vi "Report_Status_Channels.vi"(8 "error in (no error)":errorcluster, 9 "FIFO Indexes":i32[](array[numeric]), 10 "Iteration Duration (us)":u32, 11 "Data (in)":dbl[](array[numeric])) -> (0 "error out":errorcluster, 3 "Data (out)":dbl[](array[numeric]))   [LabVIEW 2019, in "Ballard Arinc-429 Engine.lvlib"]
uses:
  Ballard Arinc-429 Engine.lvlib
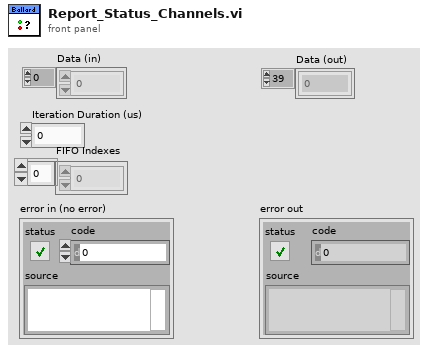
[diagram p1: front panel]
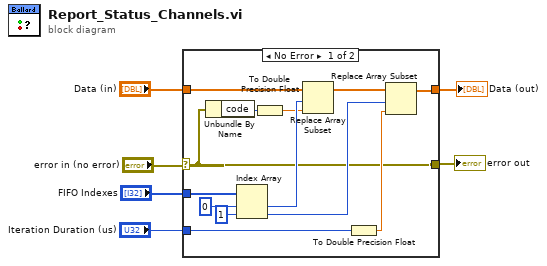
[diagram p0: block diagram]
diagram:
  n1 = case shown="No Error" "error in (no error)" {
    selector: "error in (no error)" -> [w10 w21]
    tunnel: [w10 w21] -> w5
    tunnel: "Data (in)" -> [w19 w20]
    tunnel: [w13 w20] -> w3
    tunnel: "FIFO Indexes" -> [w18 _]
    tunnel: "Iteration Duration (us)" -> [w7 _]
    frame No Error {
      n2 = Unbundle By Name(w10) -> ("code"=w9:i32)
      n3 = Index Array(array=w18, index #1=0 ("index"), index #2=1 ("index")) -> (element #1=w15:i32, element #2=w12:i32)
      n4 = To Double Precision Float(number=w9) -> (double precision float=w8:dbl)
      n5 = Replace Array Subset(array=w19, new element=w8, index=w15) -> (w14:dbl[])
      n6 = To Double Precision Float(number=w7) -> (double precision float=w11:dbl)
      n7 = Replace Array Subset(array=w14, new element=w11, index=w12) -> (w13:dbl[])
    }
    frame Error {
    }
  }
  "error out" <- w5
  "Data (out)" <- w3
